vi "Get Ball By Camera.vi"(7 "Camera":i16=1) -> (4 "Field Relative X":dbl, 6 "Robot Relative X":dbl, 8 "Robot Relative Y":dbl, 10 "Camera Relative X":dbl, 14 "Ball Found?":bool, 15 "Camera Relative Y":dbl)   [LabVIEW 2013]
uses:
  Robot Global Data.vi
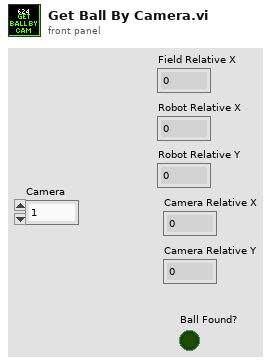
[diagram p1: front panel]
types:
  T1 = typedef "Vision Packet.ctl" = cluster{"Ball Found?":bool, "Ball X":dbl, "Ball Y":dbl, "Ball Diameter":dbl, "Gyro":dbl, "Vision Target":T2, "Timestamp":u32, "Camera":i16}
  T2 = typedef "Goal Info.ctl" = cluster{"Found?":bool, "Target Center":cluster{"X":dbl, "Y":dbl}, "Distance (ft)":dbl, "Hot?":bool, "Width":dbl, "Left?":bool}
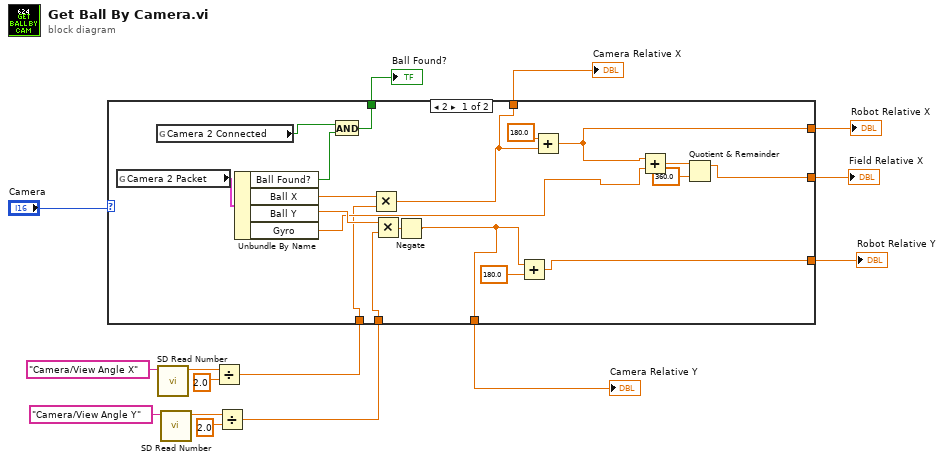
[diagram p0: block diagram]
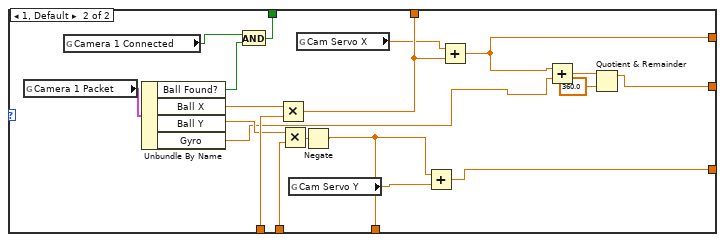
[diagram p2: hidden frame]
diagram:
  n1 = call <vilib>:"SD Read Number.vi"("Name"="Camera/View Angle X") -> ("Numeric"=w11:dbl)  [unwired: 8 in, 2 out]
  n2 = call <vilib>:"SD Read Number.vi"("Name"="Camera/View Angle Y") -> ("Numeric"=w14:dbl)  [unwired: 8 in, 2 out]
  n3 = Divide(x=w11, y=2.0) -> (x/y=w9:dbl)
  n4 = Divide(x=w14, y=2.0) -> (x/y=w8:dbl)
  n5 = case shown="2" "Camera" {
    tunnel: w9 -> [w24 w51]
    tunnel: w8 -> [w23 w49]
    tunnel: [w22 w47] -> w7
    tunnel: [w17 w45] -> w6
    tunnel: [w20 w44] -> w5
    tunnel: [w16 w43] -> w4
    tunnel: [w25 w39] -> w3
    tunnel: [w19 w35] -> w2
    frame 2 {
      n6 = global read "Robot Global Data.vi" "Camera 2 Packet"() -> (w34:T1)
      n7 = global read "Robot Global Data.vi" "Camera 2 Connected"() -> (w29:bool)
      n8 = Unbundle By Name(w34) -> ("Ball Found?"=w30:bool, "Ball X"=w33:dbl, "Ball Y"=w32:dbl, "Gyro"=w28:dbl)
      n9 = And(x=w29, y=w30) -> (x .and. y?=w25:bool)
      n10 = Multiply(x=w33, y=w24) -> (x*y=w22:dbl)
      n11 = Multiply(x=w32, y=w23) -> (x*y=w31:dbl)
      n12 = Negate(x=w31) -> (-x=w16:dbl)
      n13 = Add(x=w16, y=180.0) -> (x+y=w17:dbl)
      n14 = Add(x=180.0, y=w22) -> (x+y=w20:dbl)
      n15 = Add(x=w20, y=w28) -> (x+y=w27:dbl)
      n16 = Quotient & Remainder(x=w27, y=360.0) -> (x-y*floor(x/y)=w19:dbl)  [unwired: 1 out]
    }
    frame 1, Default {
      n17 = global read "Robot Global Data.vi" "Camera 1 Packet"() -> (w53:T1)
      n18 = global read "Robot Global Data.vi" "Camera 1 Connected"() -> (w40:bool)
      n19 = Unbundle By Name(w53) -> ("Ball Found?"=w41:bool, "Ball X"=w52:dbl, "Ball Y"=w50:dbl, "Gyro"=w38:dbl)
      n20 = And(x=w40, y=w41) -> (x .and. y?=w39:bool)
      n21 = Multiply(x=w52, y=w51) -> (x*y=w47:dbl)
      n22 = Multiply(x=w50, y=w49) -> (x*y=w42:dbl)
      n23 = global read "Robot Global Data.vi" "Cam Servo Y"() -> (w48:dbl)
      n24 = global read "Robot Global Data.vi" "Cam Servo X"() -> (w46:dbl)
      n25 = Negate(x=w42) -> (-x=w43:dbl)
      n26 = Add(x=w43, y=w48) -> (x+y=w45:dbl)
      n27 = Add(x=w46, y=w47) -> (x+y=w44:dbl)
      n28 = Add(x=w44, y=w38) -> (x+y=w37:dbl)
      n29 = Quotient & Remainder(x=w37, y=360.0) -> (x-y*floor(x/y)=w35:dbl)  [unwired: 1 out]
    }
  }
  "Robot Relative X" <- w5
  "Robot Relative Y" <- w6
  "Camera Relative X" <- w7
  "Camera Relative Y" <- w4
  "Field Relative X" <- w2
  "Ball Found?" <- w3
